vi "OpenSF.vi"() -> (0 "error out":errorcluster, 1 "read buffer 5":string, 2 "connection ID":refnum<k5>)   [LabVIEW 2011]
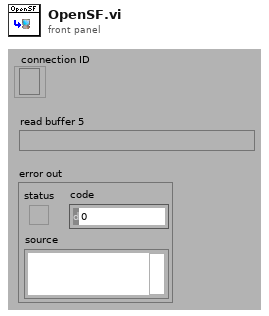
[diagram p1: front panel]
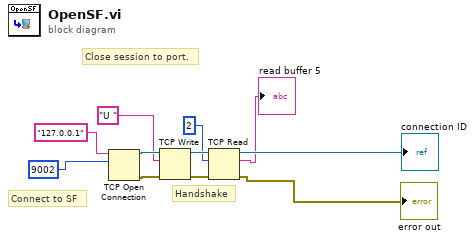
[diagram p0: block diagram]
diagram:
  # "Handshake"
  # "Connect to SF"
  # "Close session to port."
  n1 = TCP Open Connection(address="127.0.0.1", remote port or service name=9002) -> (connection ID=w5:refnum<k5>, error out=w4:errorcluster)  [unwired: 3 in]
  n2 = TCP Write(connection ID=w5, data in="U ", error in (no error)=w4) -> (connection ID out=w6:refnum<k5>, error out=w7:errorcluster)  [unwired: 1 in, 1 out]
  n3 = TCP Read(connection ID=w6, bytes to read=2, error in (no error)=w7) -> (connection ID out=→"connection ID":refnum<k5>, data out=→"read buffer 5":string, error out=→"error out":errorcluster)  [unwired: 2 in]
